vi "SetDisplayTextState.vi"(8 "Error In":errorcluster, 9 "Enabled?":bool, 10 "Window":u8=1 min=1 max=2 step=1, 11 "Keithley 6482 In":refnum<visa-resource-name>) -> (0 "Error Out":errorcluster, 3 "Keithley 6482 Out":refnum<visa-resource-name>)   [LabVIEW 2014, in "Keithley-6482-Visa.lvlib"]
uses:
  Keithley-6482-Visa.lvlib
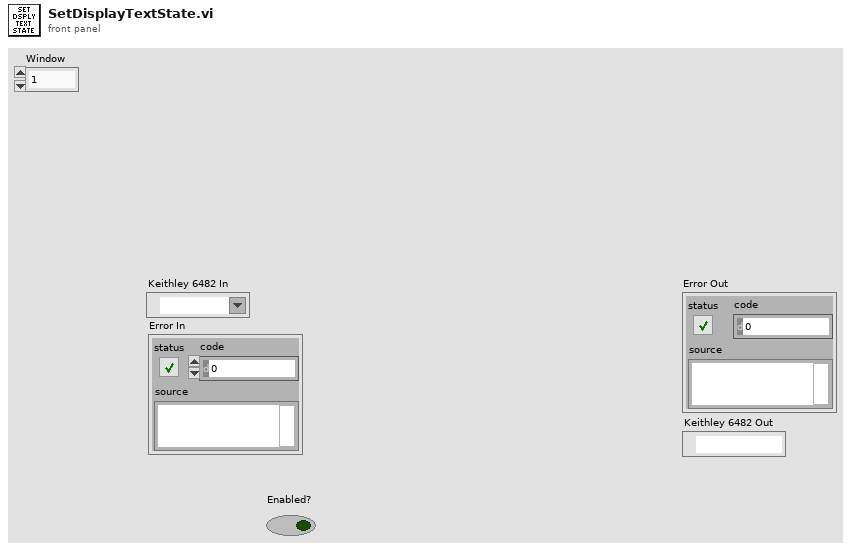
[diagram p1: front panel]
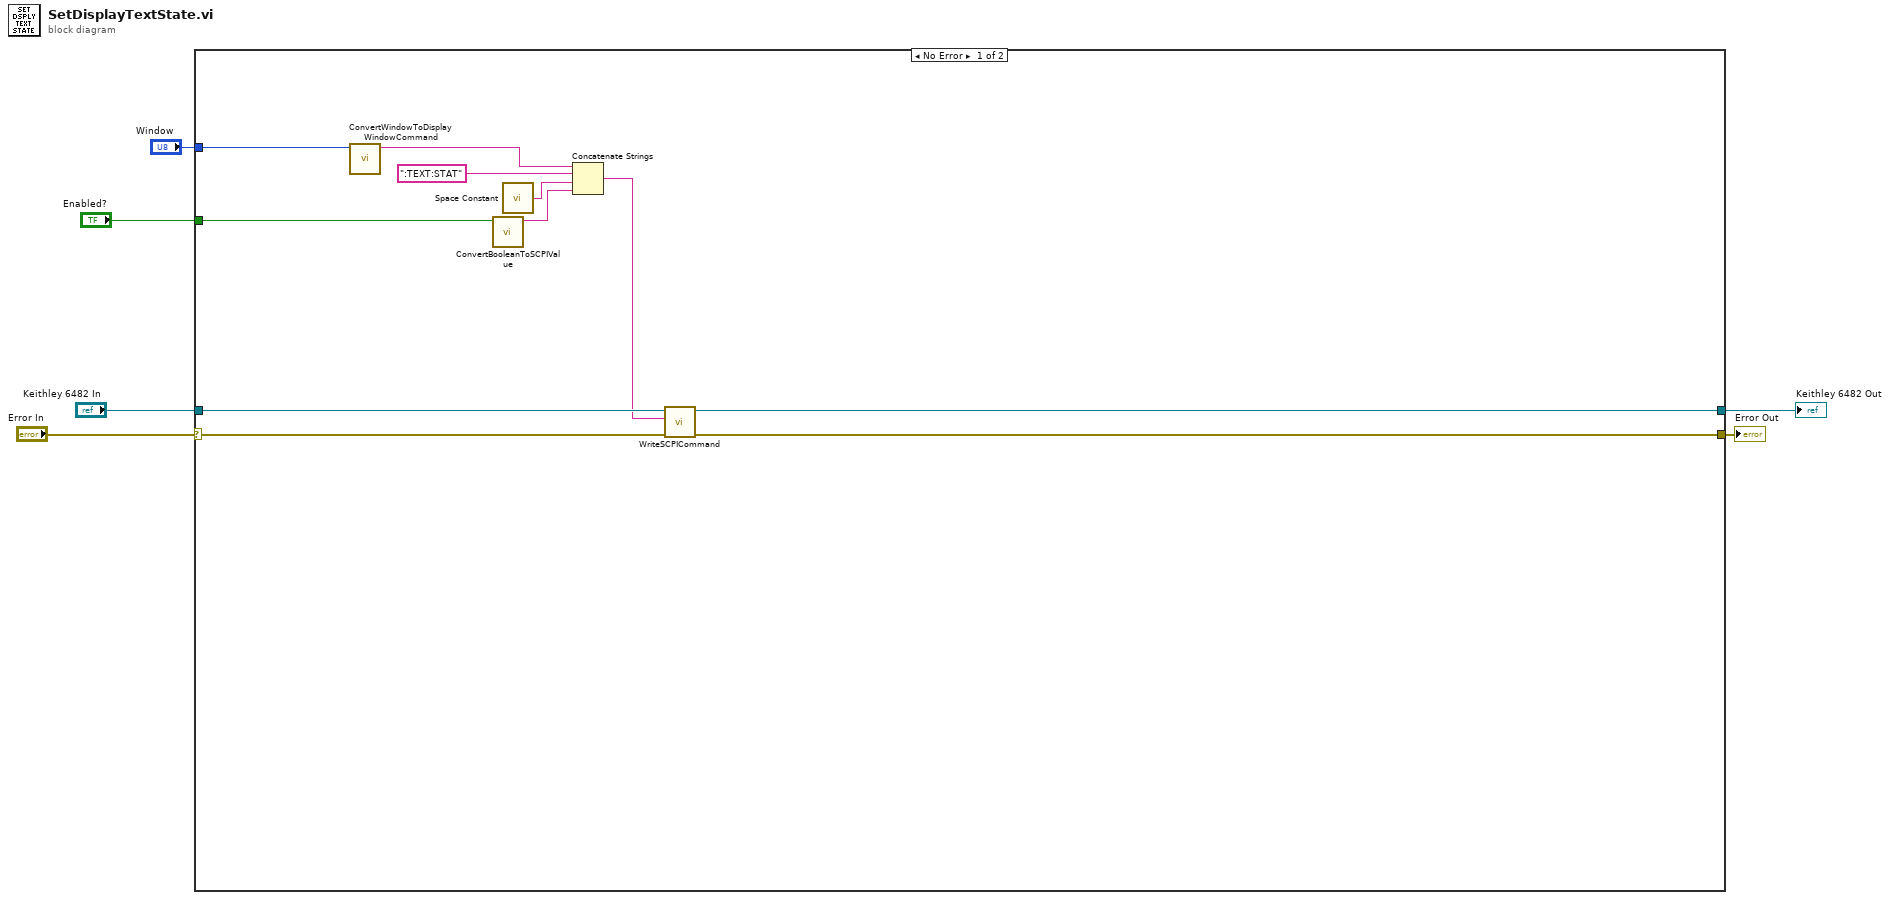
[diagram p0: block diagram]
diagram:
  n1 = case shown="No Error" "Error In" {
    selector: "Error In" -> [w10 w18]
    tunnel: "Keithley 6482 In" -> [w13 w19]
    tunnel: [w11 w18] -> w4
    tunnel: [w12 w19] -> w3
    tunnel: "Enabled?" -> [w17 _]
    tunnel: "Window" -> [w7 _]
    frame No Error {
      n2 = call "ConvertWindowToDisplayWindowCommand.vi"("Window"=w7) -> ("Display Window Command"=w8:string)  [unwired: 10 in]
      n3 = call "ConvertBooleanToSCPIValue.vi"("Boolean"=w17) -> ("SCPI Value"=w14:string)  [unwired: 10 in]
      n4 = call <vilib>:"Space Constant.vi"() -> ("String"=w15:string)
      n5 = Concatenate Strings(w8, ":TEXT:STAT", w15, w14) -> (w9:string)
      n6 = call "WriteSCPICommand.vi"("Error In"=w10, "SCPI Command"=w9, "Keithley 6482 In"=w13) -> ("Error Out"=w11:errorcluster, "Keithley 6482 Out"=w12:refnum<visa-resource-name>)  [unwired: 7 in]
    }
    frame Error {
    }
  }
  "Error Out" <- w4
  "Keithley 6482 Out" <- w3
